vi "Zoom.vi"() -> ()   [LabVIEW 2014]
doc: "Use this template to build a VI to use as a subVI."
uses:
  <vilib>/vision/NI_Vision_Development_Module.lvlib
panel:
  out "Img Display":T1(plugin-control)
  # ":: MVi Framework V1.0 ::\nAuthor:Gaoke Yang\nEmail: gaoke.yang@yahoo.com\nWeb: www.mvicontrol.com\nCopyright (C) 2015, MVI Technologies All Rights Reserved"
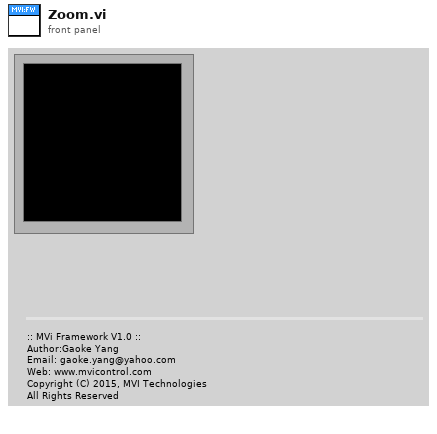
[diagram p1: front panel]
types:
  T1 = typedef "IMAQ Image.ctl" = refnum<image>
  T2 = typedef "Image Type" = u32
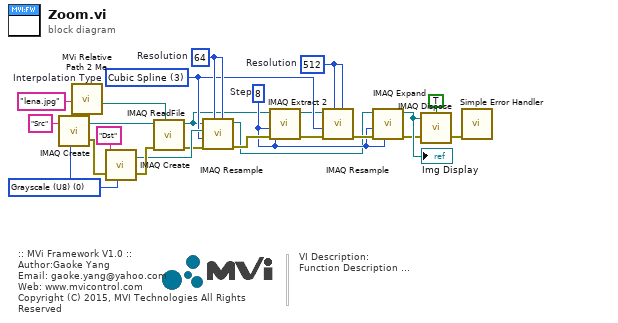
[diagram p0: block diagram]
diagram:
  w8 = 512  # Resolution
  w6 = 8  # Step
  w9 = 64  # Resolution
  w7 = u32 3 items=["Zero Order", "Bi-Linear", "Quadratic", "Cubic Spline"]  # Interpolation Type
  w18 = T2 0 items=["Grayscale (U8)", "Grayscale (I16)", "Grayscale (SGL)", "Complex (CSG)", "RGB (U32)", "HSL (U32)", "RGB (U64)", "Grayscale (U16)"] ("Image Type")
  # "VI Description:\nFunction Description ..."
  # ":: MVi Framework V1.0 ::\nAuthor:Gaoke Yang\nEmail: gaoke.yang@yahoo.com\nWeb: www.mvicontrol.com\nCopyright (C) 2015, MVI Technologies All Rights Reserved"
  n1 = call "IMAQ Create"("Image Name"="Src" ("name or relative path"), "Image Type"=w18) -> ("New Image"=w15:T1, "error out"=w17:errorcluster)  [unwired: 2 in, 1 out]
  n2 = call "MVi Relative Path 2 Me.vi"("Relative Path"="lena.jpg" ("name or relative path")) -> ("Appended Dir"=w20:path)  [unwired: 5 in, 1 out]
  n3 = call "IMAQ Create"("Image Name"="Dst" ("name or relative path"), "Image Type"=w18, "error in (no error)"=w17) -> ("New Image"=w14:T1, "error out"=w16:errorcluster)  [unwired: 1 in, 1 out]
  n4 = call "IMAQ ReadFile"("File Path"=w20, "error in (no error)"=w16, "Image"=w15) -> ("error out"=w13:errorcluster, "Image Out"=w5:T1)  [unwired: 4 in, 3 out]
  n5 = call "IMAQ Resample"("X Resolution"=w9, "Y Resolution"=w9, "error in (no error)"=w13, "Interpolation Type"=w7, "Image Dst"=w14, "Image Src"=w5) -> ("error out"=w12:errorcluster, "Image Dst Out"=w3:T1)  [unwired: 4 in]
  n6 = call "IMAQ Extract 2"("Y Step Size"=w6, "error in (no error)"=w12, "X Step Size"=w6, "Image Src"=w5) -> ("error out"=w10:errorcluster, "Image Dst Out"=w4:T1)  [unwired: 6 in]
  n7 = call "IMAQ Resample"("X Resolution"=w8, "Y Resolution"=w8, "error in (no error)"=w10, "Interpolation Type"=w7, "Image Src"=w4) -> ("error out"=w11:errorcluster)  [unwired: 5 in, 1 out]
  n8 = call "IMAQ Expand"("Y Duplication Step"=w6, "error in (no error)"=w11, "X Duplication Step"=w6, "Image Src"=w3) -> ("error out"=w1:errorcluster, "Image Dst Out"=w2:T1)  [unwired: 6 in]
  "Img Display" <- w2
  n9 = call "IMAQ Dispose"("All Images? (No)"=TRUE, "Image"=w2, "error in (no error)"=w1) -> ("error out"=w21:errorcluster)  [unwired: 3 out]
  n10 = call <vilib>:"Simple Error Handler.vi"("error in (no error)"=w21) -> ()  [unwired: 1 in, 8 out]
